vi "core_ms2s.vi"(2 "ms":i32) -> (7 "s":dbl format="%#_13g")   [LabVIEW 2015]
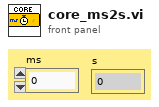
[diagram p1: front panel]
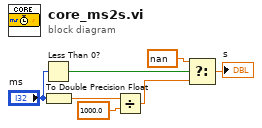
[diagram p0: block diagram]
diagram:
  n1 = Less Than 0?(x="ms") -> (x < 0?=w7:bool)
  n2 = To Double Precision Float(number="ms") -> (double precision float=w5:dbl)
  n3 = Divide(x=w5, y=1000.0) -> (x/y=w2:dbl)
  n4 = Select(t=nan ("s? t:f"), s=w7, f=w2) -> (s? t:f=→"s":dbl)
